vi "S2C_ExeScriptProcess.vi"(8 "Error In":errorcluster) -> (0 "Error Out":errorcluster, 2 "Measurement":string)   [LabVIEW 2015]
doc: "Updates the execution table results cell to \"Testing\" and performs all associated line item actions."
uses:
  Controls/S2C_ResultStatus.ctl
  Globals/S2C_Globals.vi
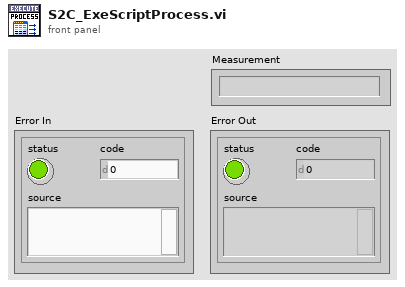
[diagram p1: front panel]
types:
  T1 = typedef "S2C_ResultStatus.ctl" = enum16{"Passed", "Failed", "Logged", "Aborted", "Error", "Testing...", "Paused", "No Record"}
  T2 = cluster{"Driver":string, "Command":string, "Return":string, "Parameters":string, "Timeout":dbl}
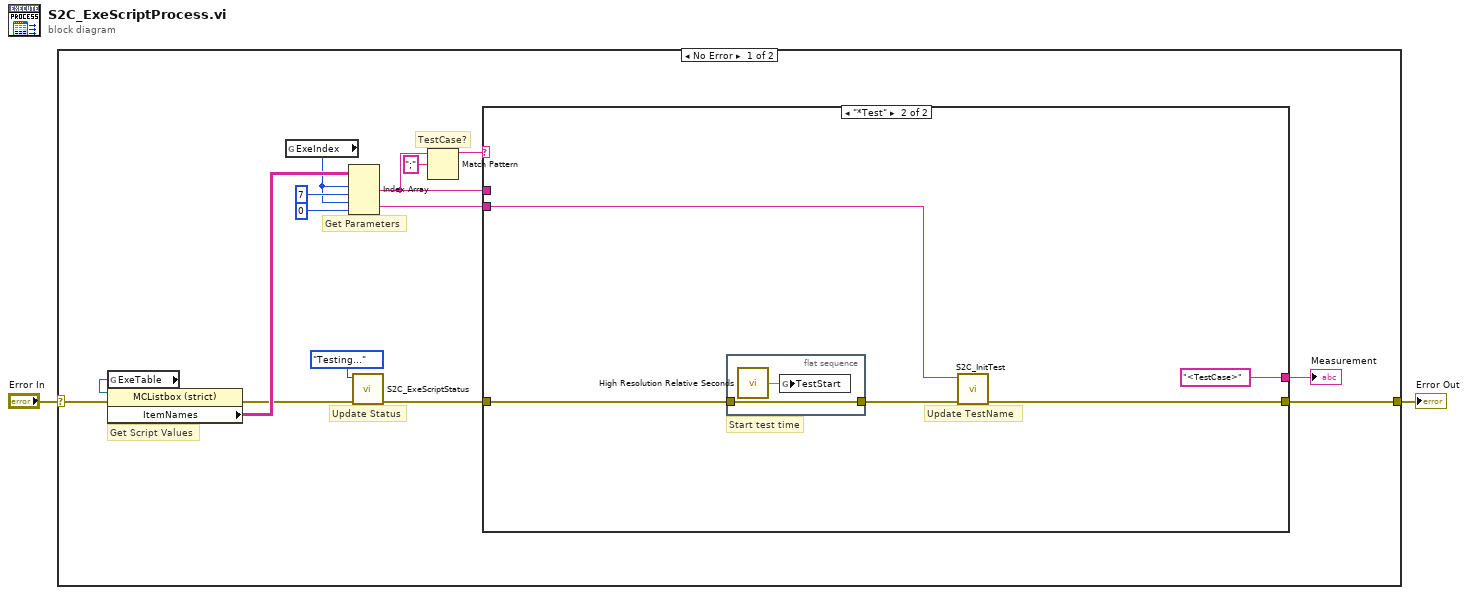
[diagram p0: block diagram]
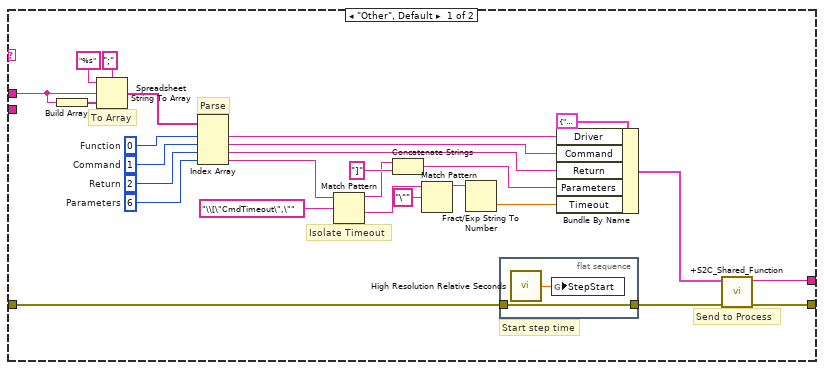
[diagram p2: hidden frame]
diagram:
  n1 = case shown="No Error" "Error In" {
    selector: "Error In" -> [w4 w54]
    tunnel: [w6 w54] -> w1
    frame No Error {
      # "Get Script Values"
      # "Update Status"
      # "TestCase?"
      # "Get Parameters"
      n2 = global read "S2C_Globals.vi" "ExeTable"() -> (w3:refnum<vi>)
      n3 = property class="MCListbox (strict)"(reference=w3, error in=w4) -> (error out=w8:errorcluster, "ItemNames"=w17:string[][])  [unwired: 1 out]
      n4 = global read "S2C_Globals.vi" "ExeIndex"() -> (w14:i32)
      n5 = Index Array(array=w17, index (row) #1=w14, index (col) #1=7 ("disabled index (col)"), index (row) #2=w14, index (col) #2=0 ("disabled index (col)")) -> (element #1=w12:string, element #2=w9:string)
      n6 = call "S2C_ExeScriptStatus.vi"("Error In"=w8, "Status"=S2C_ResultStatus."Testing...") -> ("Error Out"=w7:errorcluster)  [unwired: 9 in]
      n7 = Match Pattern(string=w12, regular expression=";") -> (before substring=w10:string)  [unwired: 1 in, 3 out]
      n8 = case shown="\"*Test\"" w10 {
        tunnel: w7 -> [w19 w47]
        tunnel: [w44 "<TestCase>" ("Response")] -> w16
        tunnel: [w20 w48] -> w6
        tunnel: w12 -> [w39 _]
        tunnel: w9 -> [_ w50]
        frame "Other", Default {
          w33 = 6  # Parameters
          w34 = 2  # Return
          w35 = 1  # Command
          w36 = 0  # Function
          # "Start step time"
          # "Parse"
          # "To Array"
          # "Send to Process"
          # "Isolate Timeout"
          n9 = Build Array(w39) -> (w38:string[])
          n10 = Spreadsheet String To Array(delimiter (Tab)=";", format string="%s", spreadsheet string=w39, array type (2D Dbl)=w38) -> (array=w37:string[])
          n11 = Index Array(array=w37, index #1=w36, index #2=w35, index #3=w34, index #4=w33) -> (element #1=w30:string, element #2=w31:string, element #3=w32:string, element #4=w23:string)
          n12 = Match Pattern(string=w23, regular expression="\\[\"CmdTimeout\",\"") -> (before substring=w24:string, after substring=w28:string)  [unwired: 1 in, 2 out]
          n13 = Concatenate Strings(w24, "]" ("string")) -> (w22:string)
          n14 = Match Pattern(string=w28, regular expression="\"") -> (before substring=w26:string)  [unwired: 1 in, 3 out]
          n15 = Fract/Exp String To Number(string=w26) -> (number=w21:dbl)  [unwired: 3 in, 1 out]
          n16 = flat-sequence {
            tunnel: w19 -> [w45]
            tunnel: [w45] -> w18
            frame #0 {
              n17 = call <vilib>:"High Resolution Relative Seconds.vi"() -> ("relative seconds"=w46:dbl)
              n18 = global write "S2C_Globals.vi" "StepStart"(w46) -> ()
            }
          }
          n19 = Bundle By Name(cluster=T2 {"Driver"="", "Command"="", "Return"="", "Parameters"="", "Timeout"=0.0}, "Driver"=w30, "Command"=w31, "Return"=w32, "Parameters"=w22, "Timeout"=w21) -> (w42:T2)
          n20 = call "+S2C_Shared_Function.vi"("Error In"=w18, "Settings"=w42) -> ("Error Out"=w20:errorcluster, "Response"=w44:string)  [unwired: 8 in]
        }
        frame "*Test" {
          # "Start test time"
          # "Update TestName"
          n21 = flat-sequence {
            tunnel: w47 -> [w52]
            tunnel: [w52] -> w49
            frame #0 {
              n22 = call <vilib>:"High Resolution Relative Seconds.vi"() -> ("relative seconds"=w53:dbl)
              n23 = global write "S2C_Globals.vi" "TestStart"(w53) -> ()
            }
          }
          n24 = call "S2C_InitTest.vi"("Error In"=w49, "TestName"=w50) -> ("Error Out"=w48:errorcluster)  [unwired: 9 in]
        }
      }
      "Measurement" <- w16
    }
    frame Error {
    }
  }
  "Error Out" <- w1
